vi "Get Name.vi"(8 "error in (no error)":errorcluster, 11 "Not Connected in":refnum<class "Not Connected.lvclass">) -> (0 "error out":errorcluster, 2 "Name":string, 3 "Not Connected out":refnum<class "Not Connected.lvclass">)   [LabVIEW 2013, in "Receiver.lvlib" / "Not Connected.lvclass"]
uses:
  Not Connected.lvclass
  Receiver.lvclass
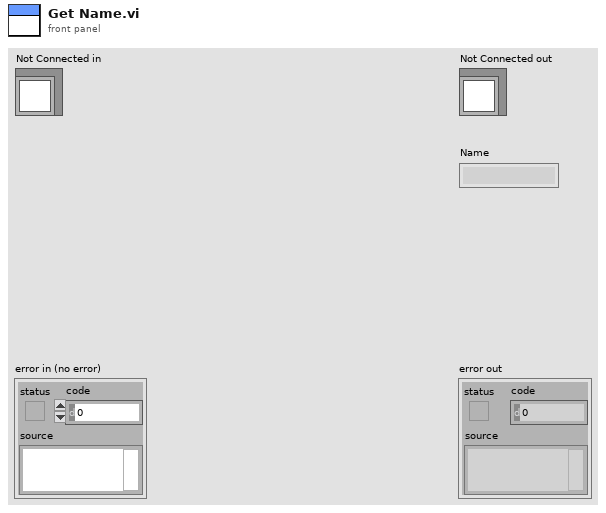
[diagram p1: front panel]
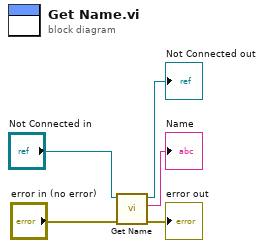
[diagram p0: block diagram]
diagram:
  n1 = call-parent "Get Name.vi"("error in (no error)"="error in (no error)", "Receiver in"="Not Connected in") -> ("error out"=→"error out":errorcluster, "Name"=→"Name":string, "Receiver out"=→"Not Connected out":refnum<class "Not Connected.lvclass">)  [unwired: 7 in]
